vi "Server.vi"() -> ()   [LabVIEW 2011]
uses:
  ATE_Machine_Status.ctl
  <vilib>/Platform/TimedLoop/XDataNode/nitl_modes.ctl
  <vilib>/Platform/TimedLoop/XDataNode/timing_clust.ctl
  <vilib>/Platform/TimedLoop/XDataNode/wakeup.ctl
  ATE_Balance_Data.ctl
  ATE_Fan_Data.ctl
  ATE_Fan_Control.ctl
  ATE_Road_Control.ctl
  ATE_Road_Data.ctl
  <vilib>/Platform/TimedLoop/XDataNode/XDataNode.xnode
  <vilib>/Platform/TimedLoop/XDataNode/XDNodeRunTimeDep.lvlib
panel:
  out "BL Suction Fan 1":i32
  out "BL Suction Fan 2":i32
  out "Road Active?":bool
  out "Set Yaw Angle":dbl
  out "Atmos Pressure":dbl
  out "Loop Status":T1 {"Poor Loops" format="%0.2f %"; "Loop Frequency" format="%0.2f Hz"}
  in  "Stop Button":bool
  out "DLL Path":path
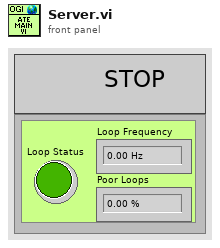
[diagram p1: front panel]
types:
  T1 = typedef "ATE_Machine_Status.ctl" = cluster{"Loop Status":bool, "Loop Frequency":dbl, "Poor Loops":dbl}
  T2 = typedef "XDNodeRunTimeDep.lvlib/nitl_modes.ctl" = enum32{"No Change", "Process missed periods, maintain original phase", "Discard missed periods, maintain original phase", "Process missed periods, ignore original phase", "Discard missed periods, ignore original phase"}
  T3 = typedef "ATE_Balance_Data.ctl" = cluster{"%Lift":dbl, "Lift":dbl, "%Pitch":dbl, "Pitch":dbl, "%Drag":dbl, "Drag":dbl, "%Side":dbl, "Side":dbl, "%Yaw":dbl, "Yaw":dbl, "%Roll":dbl, "Roll":dbl}
  T4 = typedef "ATE_Road_Data.ctl" = cluster{"Road Information":string, "Road Status":string, "Yaw Angle":dbl, "Road Speed":dbl}
  T5 = typedef "XDNodeRunTimeDep.lvlib/timing_clust.ctl" = cluster{"Expected End [f-1]":u64, "Actual End [f-1]":u64, "Finished Late? [f-1]":bool, "Expected End [i-1]":u64, "Actual End [i-1]":u64, "Finished Late? [i-1]":bool, "Expected Start [i]":u64, "Actual Start [i]":u64, "Expected Start [f]":u64, "Actual Start [f]":u64, "Source Name":string, "Structure Name":string, "Period":i64, "Deadline":i64, "Offset":i64, "Start":i64, "Priority":i32, "Timeout":i32, "Mode":T2, "Wakeup Reason":T6, "Error":errorcluster, "Source Type":string, "Secondary Source Type":string, "Global End Time":u64, "Global Start Time":u64, "Frame Duration":u64, "Iteration Duration":u64, "Assigned CPU":i32, "I/O Scan Engine Mode":u32}
  T6 = typedef "XDNodeRunTimeDep.lvlib/wakeup.ctl" = enum32{"Normal", "Aborted", "Asynchronous wakeup", "Timing source error", "Timed loop error", "Timeout"}
  T7 = typedef "ATE_Fan_Data.ctl" = cluster{"Fan Speed (RPM)":dbl, "Wind Speed (m/s)":dbl, "SMAD Data":string}
  T8 = typedef "ATE_Fan_Control.ctl" = cluster{"Reset Pitot?":bool, "Set Fan State":bool, "Set Pressure":dbl, "Set Fan Speed":dbl, "Set Wind Speed Ratio":dbl, "Tweak Change?":bool, "Speed Change?":bool}
  T9 = typedef "ATE_Road_Control.ctl" = cluster{"Sync to Wind":bool, "Start Drive":bool, "Stop Drive":bool, "BL Suction Fan 1":i32, "BL Suction Fan 2":i32, "Set Yaw Angle":dbl, "Road Active?":bool}
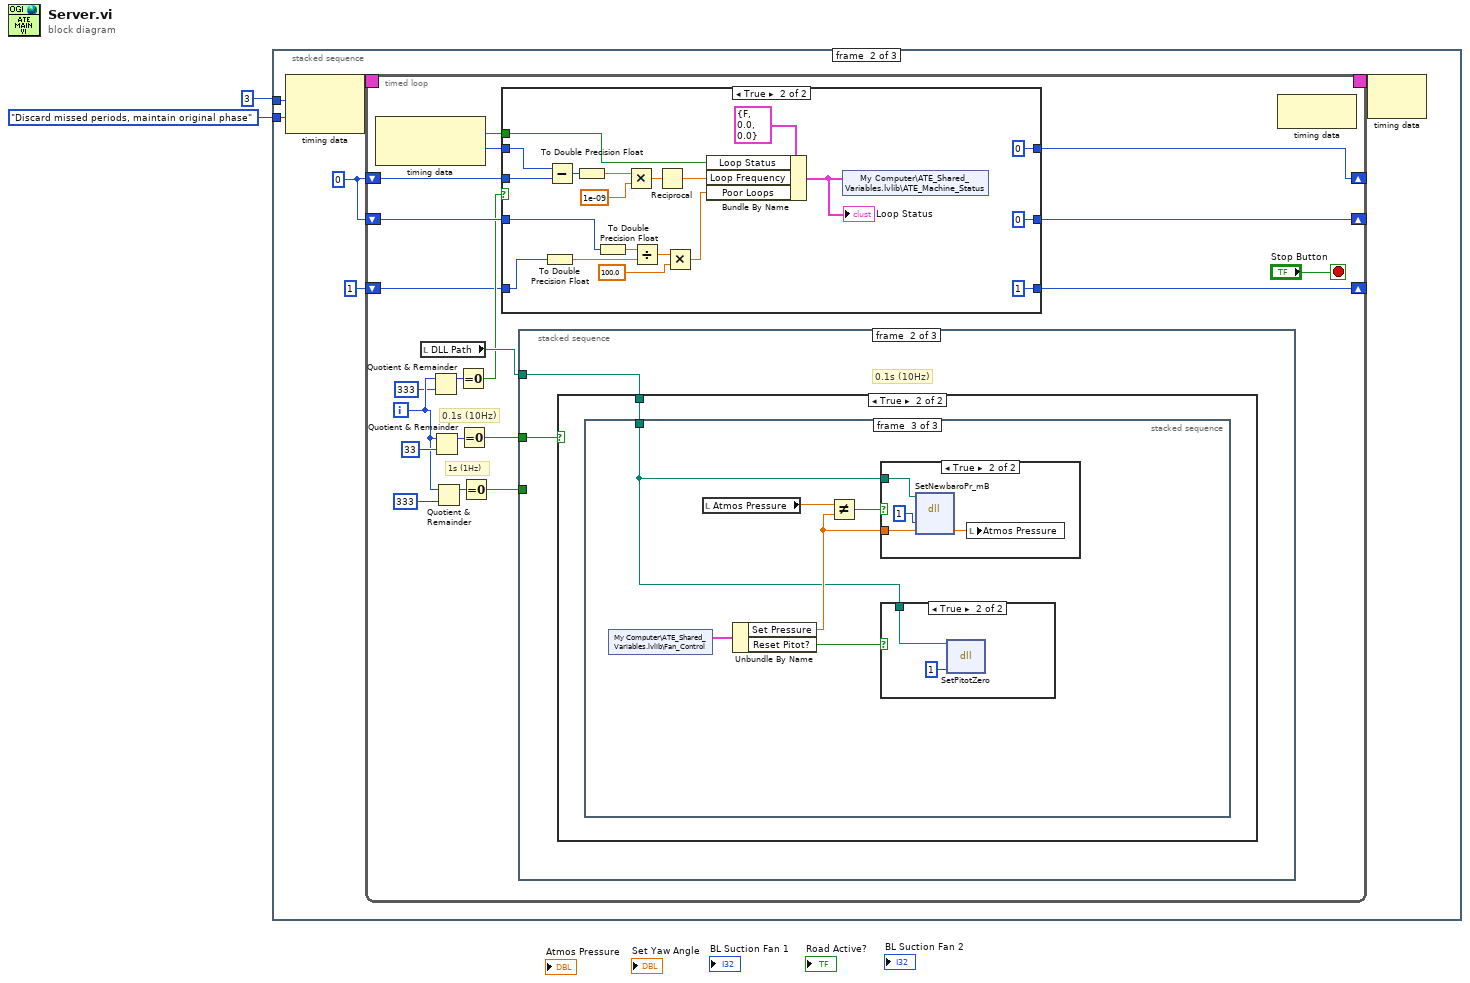
[diagram p0: block diagram]
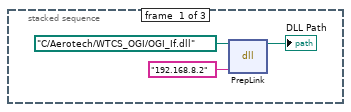
[diagram p2: hidden frame]
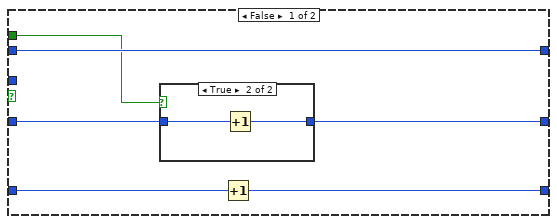
[diagram p3: hidden frame]
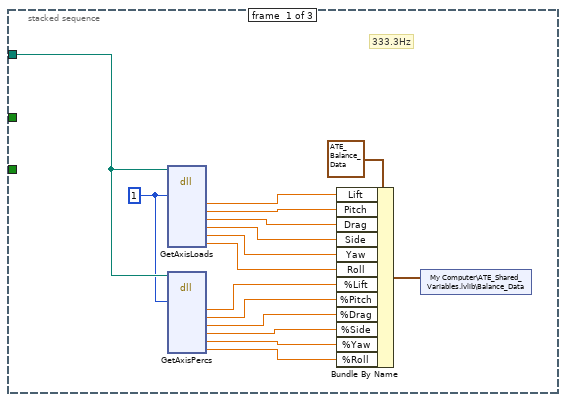
[diagram p5: hidden frame]
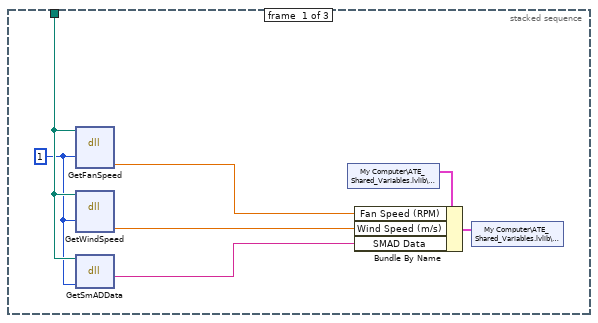
[diagram p7: hidden frame]
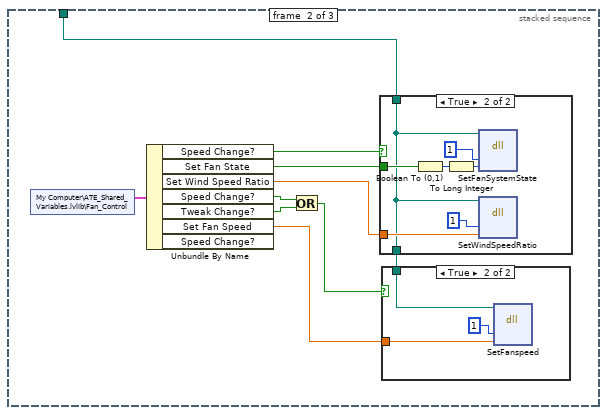
[diagram p8: hidden frame]
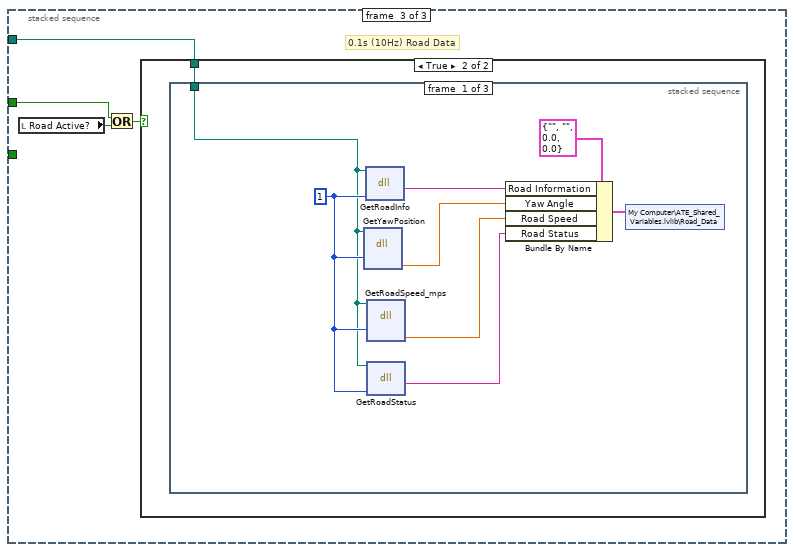
[diagram p13: hidden frame]
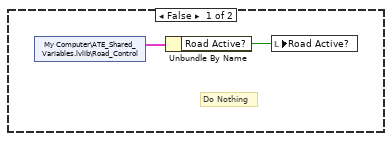
[diagram p14: hidden frame]
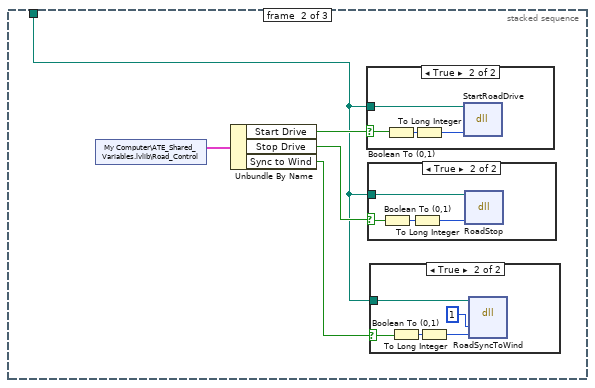
[diagram p15: hidden frame]
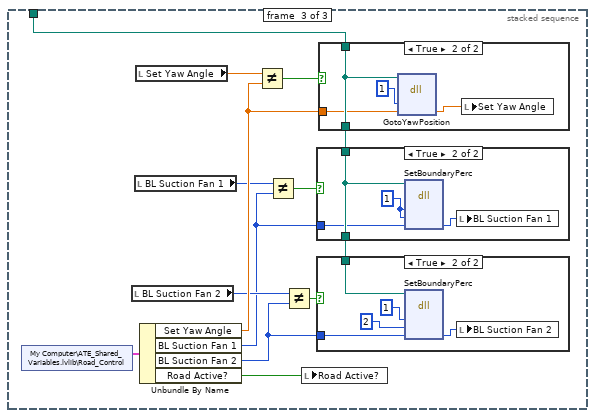
[diagram p19: hidden frame]
diagram:
  n1 = stacked-sequence {
    tunnel: nitl_modes."Discard missed periods, maintain original phase" ("Mode") -> [_ w9 _]
    tunnel: i64 3 ("Period") -> [_ w8 _]
    frame #0 {
      n2 = dll-call lib="C:/Aerotech/Drivers/OGI_IF.dll" fn="PrepLink"(path in=path "C:/Aerotech/WTCS_OGI/OGI_If.dll", "IPAddress"="192.168.8.2") -> (path out=→"DLL Path":path)  [unwired: 2 in, 3 out]
    }
    frame #1 {
      w7 = i64 0 ("Global Start Time")
      n3 = node-c288(w8, w9) -> (w11:T5)
      n4 = timed-loop {
        timing: w11 -> [_]
        timing-out: [_] -> w10
        shift-right: [w14] -> _
        shift-left: w7 -> [w29]
        shift-right: [w13] -> _
        shift-left: w7 -> [w28]
        shift-right: [w15] -> _
        shift-left: i64 1 -> [w12]
        i -> [w18]
        stop <- "Stop Button" stop-if-true
        # "1s (1Hz)"
        # "0.1s (10Hz)"
        n5 = node-c288() -> (w22:bool, w30:i64)  [unwired: 1 in]
        n6 = local read "DLL Path"() -> (w27:path)
        n7 = Quotient & Remainder(x=w18, y=333) -> (x-y*floor(x/y)=w19:i32)  [unwired: 1 out]
        n8 = Quotient & Remainder(x=w18, y=33) -> (x-y*floor(x/y)=w26:i32)  [unwired: 1 out]
        n9 = Quotient & Remainder(x=w18, y=333) -> (x-y*floor(x/y)=w25:i32)  [unwired: 1 out]
        n10 = Equal To 0?(x=w19) -> (x = 0?=w16:bool)
        n11 = Equal To 0?(x=w26) -> (x = 0?=w24:bool)
        n12 = Equal To 0?(x=w25) -> (x = 0?=w23:bool)
        n13 = case shown="True" w16 {
          tunnel: w30 -> [w36 w60]
          tunnel: w29 -> [_ w59]
          tunnel: w28 -> [w35 w45]
          tunnel: w22 -> [w34 w47]
          tunnel: [w32 i64 1] -> w15
          tunnel: w12 -> [w37 w42]
          tunnel: [w33 i64 0 ("Global Start Time")] -> w13
          tunnel: [w36 i64 0 ("Global Start Time")] -> w14
          frame False {
            n14 = case shown="True" w34 {
              tunnel: [w38 w39] -> w33
              tunnel: w35 -> [w38 w40]
              frame False {
              }
              frame True {
                n15 = Increment(x=w40) -> (x+1=w39:i64)
              }
            }
            n16 = Increment(x=w37) -> (x+1=w32:i64)
          }
          frame True {
            n17 = To Double Precision Float(number=w42) -> (double precision float=w50:dbl)
            n18 = Subtract(x=w60, y=w59) -> (x-y=w58:i64)
            n19 = To Double Precision Float(number=w58) -> (double precision float=w57:dbl)
            n20 = To Double Precision Float(number=w45) -> (double precision float=w54:dbl)
            n21 = Multiply(x=w57, y=1e-09) -> (x*y=w55:dbl)
            n22 = Divide(x=w54, y=w50) -> (x/y=w53:dbl)
            n23 = Reciprocal(x=w55) -> (1/x=w49:dbl)
            n24 = Multiply(x=w53, y=100.0) -> (x*y=w48:dbl)
            n25 = Bundle By Name(cluster=T1 {"Loop Status"=FALSE, "Loop Frequency"=0.0, "Poor Loops"=0.0} ("ATE Machine Status"), "Loop Status"=w47, "Loop Frequency"=w49, "Poor Loops"=w48) -> (w51:T1)
            "Loop Status" <- w51
            n26 = shared-variable "My Computer\\ATE_Shared_Variables.lvlib\\ATE_Machine_Status"(w51) -> ()  [unwired: 1 in, 1 out]
          }
        }
        n27 = stacked-sequence {
          tunnel: w27 -> [w76 w77 w123]
          tunnel: w24 -> [_ w78 w120]
          tunnel: w23 -> [_ _ _]
          frame #0 {
            w75 = 1 ("Enable")
            # "333.3Hz"
            n28 = dll-call lib="C:/Aerotech/Drivers/OGI_IF.dll" fn="GetAxisLoads"(path in=w76, "Enable"=w75) -> ("Lift"=w74:dbl, "Pitch"=w73:dbl, "Drag"=w72:dbl, "side"=w71:dbl, "Yaw"=w70:dbl, "Roll"=w69:dbl)  [unwired: 3 in, 9 out]
            n29 = dll-call lib="C:/Aerotech/Drivers/OGI_IF.dll" fn="GetAxisPercs"(path in=w76, "Enable"=w75) -> ("Lift"=w68:dbl, "Pitch"=w67:dbl, "Drag"=w66:dbl, "side"=w65:dbl, "Yaw"=w64:dbl, "Roll"=w63:dbl)  [unwired: 3 in, 9 out]
            n30 = Bundle By Name(cluster=T3 {"%Lift"=0.0, "Lift"=0.0, "%Pitch"=0.0, "Pitch"=0.0, "%Drag"=0.0, "Drag"=0.0, "%Side"=0.0, "Side"=0.0, "%Yaw"=0.0, "Yaw"=0.0, "%Roll"=0.0, "Roll"=0.0} ("Balance Load Data"), "Lift"=w74, "Pitch"=w73, "Drag"=w72, "Side"=w71, "Yaw"=w70, "Roll"=w69, "%Lift"=w68, "%Pitch"=w67, "%Drag"=w66, "%Side"=w65, "%Yaw"=w64, "%Roll"=w63) -> (w62:T3)
            n31 = shared-variable "My Computer\\ATE_Shared_Variables.lvlib\\Balance_Data"(w62) -> ()  [unwired: 1 in, 1 out]
          }
          frame #1 {
            # "0.1s (10Hz)"
            n32 = case shown="True" w78 {
              tunnel: w77 -> [_ w79]
              frame False {
                # "Do Nothing"
              }
              frame True {
                n33 = stacked-sequence {
                  tunnel: w79 -> [w81 w93 w108]
                  frame #0 {
                    w80 = 1 ("Enable")
                    n34 = dll-call lib="C:/Aerotech/Drivers/OGI_IF.dll" fn="GetFanSpeed"(path in=w81, "Enable"=w80) -> ("FanSpeedinRPM"=w83:dbl)  [unwired: 3 in, 4 out]
                    n35 = dll-call lib="C:/Aerotech/Drivers/OGI_IF.dll" fn="GetWindSpeed"(path in=w81, "Enable"=w80) -> ("Windspeed_M/s"=w84:dbl)  [unwired: 3 in, 4 out]
                    n36 = dll-call lib="C:/Aerotech/Drivers/OGI_IF.dll" fn="GetSmADData"(path in=w81, "Enable"=w80) -> ("SmAD Data String"=w85:string)  [unwired: 2 in, 3 out]
                    n37 = shared-variable "My Computer\\ATE_Shared_Variables.lvlib\\Fan_Data"() -> (w86:T7)  [unwired: 1 in, 1 out]
                    n38 = Bundle By Name(cluster=w86, "Fan Speed (RPM)"=w83, "Wind Speed (m/s)"=w84, "SMAD Data"=w85) -> (w82:T7)
                    n39 = shared-variable "My Computer\\ATE_Shared_Variables.lvlib\\Fan_Data"(w82) -> ()  [unwired: 1 in, 1 out]
                  }
                  frame #1 {
                    n40 = shared-variable "My Computer\\ATE_Shared_Variables.lvlib\\Fan_Control"() -> (w96:T8)  [unwired: 1 in, 1 out]
                    n41 = Unbundle By Name(w96) -> ("Speed Change?"=w94:bool, "Set Fan State"=w95:bool, "Set Wind Speed Ratio"=w92:dbl, "Speed Change?"=w90:bool, "Tweak Change?"=w89:bool, "Set Fan Speed"=w87:dbl)  [unwired: 1 out]
                    n42 = Or(x=w90, y=w89) -> (x .or. y?=w88:bool)
                    n43 = case shown="True" w94 {
                      tunnel: w95 -> [_ w105]
                      tunnel: w93 -> [w100 w103]
                      tunnel: w92 -> [_ w104]
                      tunnel: [w100 w103] -> w91
                      frame False {
                      }
                      frame True {
                        n44 = Boolean To (0,1)(Boolean=w105) -> (0, 1=w106:i16)
                        n45 = To Long Integer(number=w106) -> (32bit integer=w107:i32)
                        n46 = dll-call lib="C:/Aerotech/Drivers/OGI_IF.dll" fn="SetFanSystemState"(path in=w103, "Enable"=1, "Fan ONOFF"=w107) -> ()  [unwired: 3 in, 4 out]
                        n47 = dll-call lib="C:/Aerotech/Drivers/OGI_IF.dll" fn="SetWindSpeedRatio"(path in=w103, "Enable"=1, "Required WindSpeedRatio"=w104) -> ()  [unwired: 4 in, 3 out]
                      }
                    }
                    n48 = case shown="True" w88 {
                      tunnel: w91 -> [_ w99]
                      tunnel: w87 -> [_ w98]
                      frame False {
                      }
                      frame True {
                        n49 = dll-call lib="C:/Aerotech/Drivers/ATE_Surrey_WTCS.dll" fn="SetFanspeed"(path in=w99, "Enable"=1, "NewFanSpeed"=w98) -> ()  [unwired: 3 in, 4 out]
                      }
                    }
                  }
                  frame #2 {
                    n50 = shared-variable "My Computer\\ATE_Shared_Variables.lvlib\\Fan_Control"() -> (w113:T8)  [unwired: 1 in, 1 out]
                    n51 = local read "Atmos Pressure"() -> (w111:dbl)
                    n52 = Unbundle By Name(w113) -> ("Set Pressure"=w110:dbl, "Reset Pitot?"=w112:bool)
                    n53 = Not Equal?(x=w111, y=w110) -> (x != y?=w109:bool)
                    n54 = case shown="True" w109 {
                      tunnel: w110 -> [_ w116]
                      tunnel: w108 -> [_ w114]
                      frame False {
                      }
                      frame True {
                        n55 = dll-call lib="C:/Aerotech/Drivers/OGI_IF.dll" fn="SetNewbaroPr_mB"(path in=w114, "Enable"=1, "NewPressure"=w116) -> ("NewPressure"=w117:dbl)  [unwired: 2 in, 4 out]
                        n56 = local write "Atmos Pressure"(w117) -> ()
                      }
                    }
                    n57 = case shown="True" w112 {
                      tunnel: w108 -> [_ w118]
                      frame False {
                      }
                      frame True {
                        n58 = dll-call lib="C:/Aerotech/Drivers/OGI_IF.dll" fn="SetPitotZero"(path in=w118, "Enable"=1) -> ()  [unwired: 2 in, 4 out]
                      }
                    }
                  }
                }
              }
            }
          }
          frame #2 {
            # "0.1s (10Hz) Road Data"
            n59 = local read "Road Active?"() -> (w122:bool)
            n60 = Or(x=w120, y=w122) -> (x .or. y?=w121:bool)
            n61 = case shown="True" w121 {
              tunnel: w123 -> [_ w126]
              frame False {
                # "Do Nothing"
                n62 = shared-variable "My Computer\\ATE_Shared_Variables.lvlib\\Road_Control"() -> (w125:T9)  [unwired: 1 in, 1 out]
                n63 = Unbundle By Name(w125) -> ("Road Active?"=w124:bool)
                n64 = local write "Road Active?"(w124) -> ()
              }
              frame True {
                n65 = stacked-sequence {
                  tunnel: w126 -> [w133 w135 w166]
                  frame #0 {
                    w134 = 1 ("Enable")
                    n66 = dll-call lib="C:/Aerotech/Drivers/OGI_IF.dll" fn="GetYawPosition"(path in=w133, "Enable"=w134) -> ("Yaw Position"=w130:dbl)  [unwired: 3 in, 4 out]
                    n67 = dll-call lib="C:/Aerotech/Drivers/OGI_IF.dll" fn="GetRoadInfo"(path in=w133, "Enable"=w134) -> ("Road Info"=w129:string)  [unwired: 3 in, 2 out]
                    n68 = dll-call lib="C:/Aerotech/Drivers/OGI_IF.dll" fn="GetRoadSpeed_mps"(path in=w133, "Enable"=w134) -> ("RoadSpeed_mps"=w131:dbl)  [unwired: 3 in, 4 out]
                    n69 = dll-call lib="C:/Aerotech/Drivers/OGI_IF.dll" fn="GetRoadStatus"(path in=w133, "Enable"=w134) -> ("Road Status"=w132:string)  [unwired: 3 in, 2 out]
                    n70 = Bundle By Name(cluster=T4 {"Road Information"="", "Road Status"="", "Yaw Angle"=0.0, "Road Speed"=0.0} ("Road Data"), "Road Information"=w129, "Yaw Angle"=w130, "Road Speed"=w131, "Road Status"=w132) -> (w128:T4)
                    n71 = shared-variable "My Computer\\ATE_Shared_Variables.lvlib\\Road_Data"(w128) -> ()  [unwired: 1 in, 1 out]
                  }
                  frame #1 {
                    n72 = shared-variable "My Computer\\ATE_Shared_Variables.lvlib\\Road_Control"() -> (w139:T9)  [unwired: 1 in, 1 out]
                    n73 = Unbundle By Name(w139) -> ("Start Drive"=w138:bool, "Stop Drive"=w137:bool, "Sync to Wind"=w136:bool)
                    n74 = case shown="True" w138 {
                      selector: w138 -> [_ w150]
                      tunnel: w135 -> [_ w149]
                      frame False {
                      }
                      frame True {
                        n75 = Boolean To (0,1)(Boolean=w150) -> (0, 1=w152:i16)
                        n76 = To Long Integer(number=w152) -> (32bit integer=w151:i32)
                        n77 = dll-call lib="C:/Aerotech/Drivers/OGI_IF.dll" fn="StartRoadDrive"(path in=w149, "Enable"=w151) -> ()  [unwired: 2 in, 4 out]
                      }
                    }
                    n78 = case shown="True" w137 {
                      selector: w137 -> [_ w146]
                      tunnel: w135 -> [_ w145]
                      frame False {
                      }
                      frame True {
                        n79 = Boolean To (0,1)(Boolean=w146) -> (0, 1=w148:i16)
                        n80 = To Long Integer(number=w148) -> (32bit integer=w147:i32)
                        n81 = dll-call lib="C:/Aerotech/Drivers/OGI_IF.dll" fn="RoadStop"(path in=w145, "Enable"=w147) -> ()  [unwired: 2 in, 4 out]
                      }
                    }
                    n82 = case shown="True" w136 {
                      selector: w136 -> [_ w141]
                      tunnel: w135 -> [_ w140]
                      frame False {
                      }
                      frame True {
                        n83 = Boolean To (0,1)(Boolean=w141) -> (0, 1=w144:i16)
                        n84 = To Long Integer(number=w144) -> (32bit integer=w143:i32)
                        n85 = dll-call lib="C:/Aerotech/Drivers/OGI_IF.dll" fn="RoadSyncToWind"(path in=w140, "Enable"=1, "SynchState"=w143) -> ()  [unwired: 3 in, 4 out]
                      }
                    }
                  }
                  frame #2 {
                    n86 = shared-variable "My Computer\\ATE_Shared_Variables.lvlib\\Road_Control"() -> (w163:T9)  [unwired: 1 in, 1 out]
                    n87 = local read "BL Suction Fan 2"() -> (w156:i32)
                    n88 = local read "BL Suction Fan 1"() -> (w155:i32)
                    n89 = local read "Set Yaw Angle"() -> (w162:dbl)
                    n90 = Unbundle By Name(w163) -> ("Set Yaw Angle"=w160:dbl, "BL Suction Fan 1"=w154:i32, "BL Suction Fan 2"=w153:i32, "Road Active?"=w159:bool)
                    n91 = Not Equal?(x=w162, y=w160) -> (x != y?=w161:bool)
                    n92 = Not Equal?(x=w155, y=w154) -> (x != y?=w158:bool)
                    n93 = Not Equal?(x=w156, y=w153) -> (x != y?=w157:bool)
                    n94 = local write "Road Active?"(w159) -> ()
                    n95 = case shown="True" w161 {
                      tunnel: w166 -> [w177 w181]
                      tunnel: [w177 w181] -> w165
                      tunnel: w160 -> [_ w178]
                      frame False {
                      }
                      frame True {
                        n96 = dll-call lib="C:/Aerotech/Drivers/OGI_IF.dll" fn="GotoYawPosition"(path in=w181, "Enable"=1, "NewYawPos"=w178) -> ("NewYawPos"=w179:dbl)  [unwired: 2 in, 4 out]
                        n97 = local write "Set Yaw Angle"(w179) -> ()
                      }
                    }
                    n98 = case shown="True" w158 {
                      tunnel: w165 -> [w172 w176]
                      tunnel: [w172 w176] -> w164
                      tunnel: w154 -> [_ w174]
                      frame False {
                      }
                      frame True {
                        w175 = 1 ("enable")
                        n99 = dll-call lib="C:/Aerotech/Drivers/OGI_IF.dll" fn="SetBoundaryPerc"(path in=w176, "enable"=w175, "BL Fan (1 or 2)"=w175, "New Percentage"=w174) -> ("New Percentage"=w173:i32)  [unwired: 3 in, 4 out]
                        n100 = local write "BL Suction Fan 1"(w173) -> ()
                      }
                    }
                    n101 = case shown="True" w157 {
                      tunnel: w164 -> [_ w171]
                      tunnel: w153 -> [_ w169]
                      frame False {
                      }
                      frame True {
                        n102 = dll-call lib="C:/Aerotech/Drivers/OGI_IF.dll" fn="SetBoundaryPerc"(path in=w171, "enable"=1, "BL Fan (1 or 2)"=2 ("enable"), "New Percentage"=w169) -> ("New Percentage"=w170:i32)  [unwired: 3 in, 4 out]
                        n103 = local write "BL Suction Fan 2"(w170) -> ()
                      }
                    }
                  }
                }
              }
            }
          }
        }
        n104 = node-c288() -> ()  [unwired: 1 in, 1 out]
      }
      n105 = node-c288(w10) -> ()  [unwired: 1 out]
    }
    frame #2 {
      n106 = local read "DLL Path"() -> (w191:path)
      n107 = dll-call lib="C:/Aerotech/Drivers/OGI_IF.dll" fn="CloseLink"(path in=w191) -> ()  [unwired: 2 in, 3 out]
    }
  }
